vi "VISA wait.vi"(8 "error in (no error)":errorcluster, 11 "AOTF in":refnum<class "AOTF.lvclass">) -> (0 "error out":errorcluster, 3 "AOTF out":refnum<class "AOTF.lvclass">)   [LabVIEW 2012, in "AOTF.lvclass"]
uses:
  AOTF.lvclass
  AOTF.lvclass/AOTF.ctl
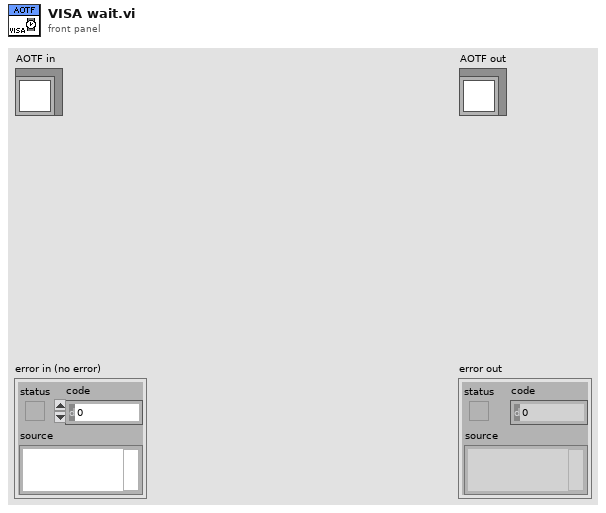
[diagram p1: front panel]
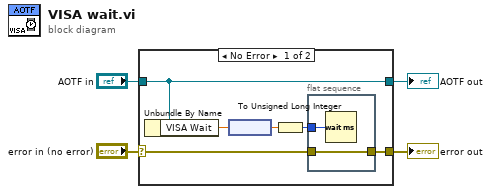
[diagram p0: block diagram]
diagram:
  n1 = case shown="No Error" "error in (no error)" {
    selector: "error in (no error)" -> [w10 w14]
    tunnel: [w9 w14] -> w3
    tunnel: [w5 w13] -> w1
    tunnel: "AOTF in" -> [w5 w13]
    frame No Error {
      n2 = Unbundle By Name(w5) -> ("VISA Wait"=w8:dbl[unit])
      n3 = node(w8) -> (w7:dbl)
      n4 = To Unsigned Long Integer(number=w7) -> (unsigned 32bit integer=w6:u32)
      n5 = flat-sequence {
        tunnel: w10 -> [w12]
        tunnel: [w12] -> w9
        tunnel: w6 -> [w11]
        frame #0 {
          n6 = Wait (ms)(milliseconds to wait=w11) -> ()  [unwired: 1 out]
        }
      }
    }
    frame Error {
    }
  }
  "error out" <- w3
  "AOTF out" <- w1
